vi "Set_Low_Speed_Video.vi"(8 "error in (no error)":errorcluster, 9 "Frame rate LS":i32, 10 "Exposure time LS":i32, 11 "Refnum in":T1) -> (0 "error out":errorcluster, 2 "ValueString":string, 3 "Refnum out":T1)   [LabVIEW 2017]
uses:
  <vilib>/userdefined/High Color/IMAQdx.ctl
  C:/Program Files (x86)/National Instruments/LabVIEW 2017/resource/objmgr/imaqdx.rc
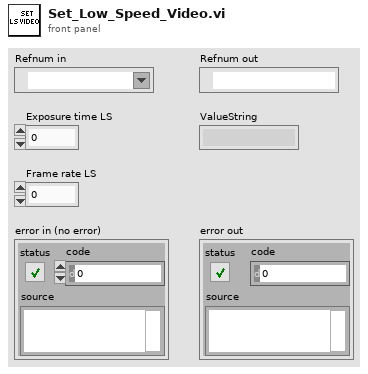
[diagram p1: front panel]
types:
  T1 = typedef "IMAQdx.ctl" = refnum<k21>
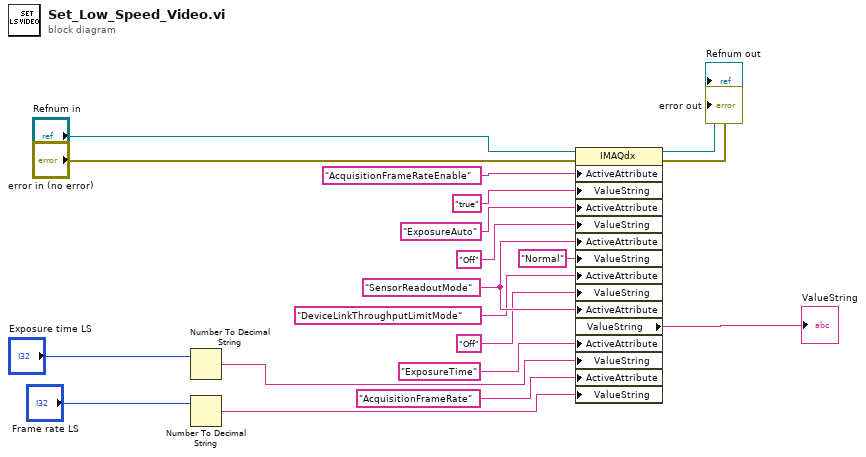
[diagram p0: block diagram]
diagram:
  w7 = "SensorReadoutMode" ("ActiveAttribute")
  n1 = Number To Decimal String(number="Exposure time LS") -> (decimal integer string=w11:string)  [unwired: 1 in]
  n2 = Number To Decimal String(number="Frame rate LS") -> (decimal integer string=w12:string)  [unwired: 1 in]
  n3 = property class="IMAQdx"(reference="Refnum in", error in="error in (no error)", "ActiveAttribute"="AcquisitionFrameRateEnable", "ValueString"="true", "ActiveAttribute"="ExposureAuto", "ValueString"="Off", "ActiveAttribute"=w7, "ValueString"="Normal", "ActiveAttribute"="DeviceLinkThroughputLimitMode", "ValueString"="Off", "ActiveAttribute"=w7, "ActiveAttribute"="ExposureTime", "ValueString"=w11, "ActiveAttribute"="AcquisitionFrameRate", "ValueString"=w12) -> (reference out=→"Refnum out":T1, error out=→"error out":errorcluster, "ValueString"=→"ValueString":string)
